vi "Obtener Path.vi"(11 "REFRESCOS Y PAPAS ACTOR in":refnum<class "REFRESCOS Y PAPAS ACTOR.lvclass">) -> (3 "appended path":path)   [LabVIEW 2019, in "REFRESCOS Y PAPAS ACTOR.lvlib" / "REFRESCOS Y PAPAS ACTOR.lvclass"]
uses:
  REFRESCOS Y PAPAS ACTOR.lvclass
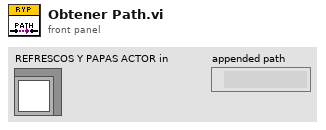
[diagram p1: front panel]
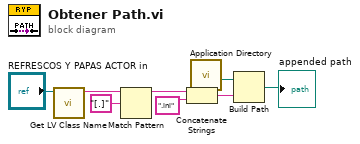
[diagram p0: block diagram]
diagram:
  n1 = call <vilib>:"Get LV Class Name.vi"("object"="REFRESCOS Y PAPAS ACTOR in") -> ("class name"=w4:string)  [unwired: 9 in, 1 out]
  n2 = Match Pattern(string=w4, regular expression="[.]") -> (before substring=w6:string)  [unwired: 1 in, 3 out]
  n3 = Concatenate Strings(w6, ".ini" ("string")) -> (w7:string)
  n4 = call <vilib>:"Application Directory.vi"() -> ("Application Directory"=w1:path)
  n5 = Build Path(base path=w1, name or relative path=w7) -> (appended path=→"appended path":path)
